vi "Periodic Tasks.vi"(8 "error in":errorcluster) -> ()   [LabVIEW 2016]
doc: "This VI runs in parallel to other tasks. It can contain as many user-defined periodic loops as you need. These can carry out PID or other sorts of timed response."
uses:
  <vilib>/Rock Robotics/SystemInterfaces/DIO/FPGA_DIOPWMChannel.ctl
  <vilib>/Rock Robotics/WPI/MotorControl/WPI_MotorControlOpen Victor.vi
  <vilib>/Rock Robotics/Network Tables/SD Write Number.vi
  <vilib>/addons/control/pid/pid.llb/PID Control Input Filter (DBL).vi
  <vilib>/addons/control/pid/pid.llb/PID (DBL).vi
  <vilib>/addons/control/pid/NI_PID_pid.lvlib
panel:
  in  "PID gains":T1={"proportional gain (Kc)"=0.1, "integral time (Ti, min)"=0.2, "derivative time (Td, min)"=0.0} {"derivative time (Td, min)" format="%.3f"; "integral time (Ti, min)" format="%.3f"; "proportional gain (Kc)" format="%.3f"}
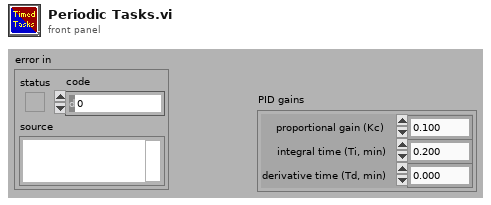
[diagram p1: front panel]
types:
  T1 = cluster{"proportional gain (Kc)":dbl, "integral time (Ti, min)":dbl, "derivative time (Td, min)":dbl}
  T2 = typedef "FPGA_DIOPWMChannel.ctl" = enum8{"PWM 0", "PWM 1", "PWM 2", "PWM 3", "PWM 4", "PWM 5", "PWM 6", "PWM 7", "PWM 8", "PWM 9", "PWM MXP 0", "PWM MXP 1", "PWM MXP 2", "PWM MXP 3", "PWM MXP 4", "PWM MXP 5", "PWM MXP 6", "PWM MXP 7", "PWM MXP 8", "PWM MXP 9", "Invalid"}
  T3 = typedef "WPI_MotorControlDeviceRef.ctl" = cluster{"DeviceStatus":errorcluster, "Type":T4, "PWM":cluster{"PWM Channel":T2, "DeadBand":T5}, "CAN":cluster{"Device Number":u8, "SetOutput VI Ref":variant, "GetOutput VI Ref":variant, "Enable VI Ref":variant, "Disable VI Ref":variant, "Data":variant}, "Invert":bool}
  T4 = typedef "WPI_MotorControlType.ctl" = enum16{"PWM", "CAN"}
  T5 = typedef "WPI_PWMDeadband.ctl" = cluster{"Name":string, "maxPositivePwm":i32, "minPositivePwm":i32, "centerPwm":i32, "maxNegativePwm":i32, "minNegativePwm":i32, "angularRange":u16}
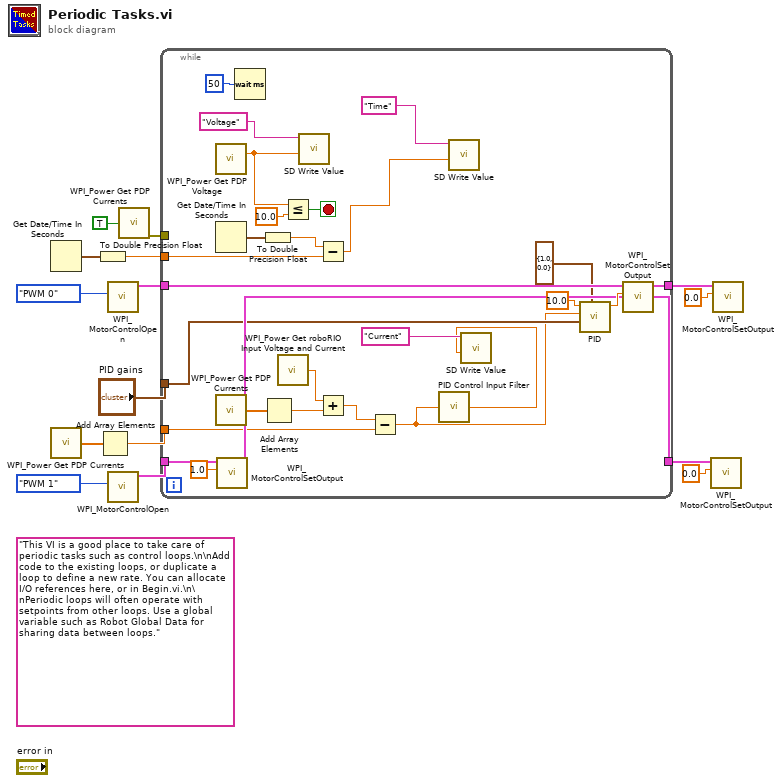
[diagram p0: block diagram]
diagram:
  (unwired) "This VI is a good place to take care of periodic tasks such as control loops.\n\nAdd code to the existing loops, or duplicate a loop to define a new rate. You can allocate I/O references here, or in Begin.vi.\n\nPeriodic loops will often operate with setpoints from other loops. Use a global variable such as Robot Global Data for sharing data between loops."
  n1 = Get Date/Time In Seconds() -> (seconds since 1Jan1904=w5:timestamp)
  n2 = call <vilib>:"WPI_Power Get PDP Currents.vi"() -> ("all currents (A)"=w2:dbl[])  [unwired: 13 in, 2 out]
  n3 = To Double Precision Float(number=w5) -> (double precision float=w4:dbl)
  n4 = Add Array Elements(numeric array=w2) -> (sum=w1:dbl)
  n5 = call-poly <vilib>:"WPI_MotorControlOpen.vi"("PWM Channel"=FPGA_DIOPWMChannel."PWM 0") -> ("MotorControlDeviceRef"=w11:T3)  [unwired: 9 in, 1 out]
  n6 = call-poly <vilib>:"WPI_MotorControlOpen.vi"("PWM Channel"=FPGA_DIOPWMChannel."PWM 1") -> ("MotorControlDeviceRef"=w10:T3)  [unwired: 9 in, 1 out]
  n7 = call <vilib>:"WPI_Power Get PDP Currents.vi"("Tare Currents?"=TRUE) -> ("error out"=w14:errorcluster)  [unwired: 12 in, 2 out]
  n8 = while {
    tunnel: w14 -> [_]
    tunnel: w11 -> [w36]
    tunnel: w10 -> [w37]
    tunnel: [w32] -> w9
    tunnel: [w31] -> w8
    tunnel: w4 -> [w27]
    tunnel: "PID gains" -> [w23]
    tunnel: w1 -> [w22]
    stop <- w33 stop-if-true
    n9 = call <vilib>:"WPI_Power Get PDP Voltage.vi"() -> ("voltage (V)"=w30:dbl)  [unwired: 14 in, 1 out]
    n10 = Get Date/Time In Seconds() -> (seconds since 1Jan1904=w29:timestamp)
    n11 = call <vilib>:"WPI_Power Get PDP Currents.vi"() -> ("all currents (A)"=w40:dbl[])  [unwired: 13 in, 2 out]
    n12 = call <vilib>:"WPI_MotorControlSetOutput.vi"("Output"=1.0, "MotorControlDevRef"=w37) -> ("MotorControlDevRef"=w31:T3)  [unwired: 7 in, 2 out]
    n13 = Wait (ms)(milliseconds to wait=u32 50) -> ()  [unwired: 1 out]
    n14 = To Double Precision Float(number=w29) -> (double precision float=w28:dbl)
    n15 = Add Array Elements(numeric array=w40) -> (sum=w38:dbl)
    n16 = call <vilib>:"WPI_Power Get roboRIO Input Voltage and Current.vi"() -> ("roboRIO input current (A)"=w39:dbl)  [unwired: 13 in, 2 out]
    n17 = Less Or Equal?(x=w30, y=10.0) -> (x <= y?=w33:bool)
    n18 = call-poly <vilib>:"SD Write Value.vi"("Numeric"=w30, "Name"="Voltage") -> ()  [unwired: 8 in, 2 out]
    n19 = Subtract(x=w28, y=w27) -> (x-y=w17:dbl)
    n20 = Add(x=w39, y=w38) -> (x+y=w21:dbl)
    n21 = Subtract(x=w21, y=w22) -> (x-y=w19:dbl)
    n22 = call-poly <vilib>:"PID Control Input Filter.vi"("input"=w19) -> ("output"=w18:dbl)  [unwired: 4 in]
    n23 = call-poly <vilib>:"SD Write Value.vi"("Numeric"=w17, "Name"="Time") -> ()  [unwired: 8 in, 2 out]
    n24 = call-poly <vilib>:"SD Write Value.vi"("Numeric"=w18, "Name"="Current") -> ()  [unwired: 8 in, 2 out]
    n25 = call-poly <vilib>:"PID.vi"("output range"=cluster{"output high":dbl, "output low":dbl} {"output high"=1.0, "output low"=0.0}, "PID gains"=w23, "process variable"=w19, "setpoint"=10.0) -> ("output"=w35:dbl)  [unwired: 6 in, 1 out]
    n26 = call <vilib>:"WPI_MotorControlSetOutput.vi"("Output"=w35, "MotorControlDevRef"=w36) -> ("MotorControlDevRef"=w32:T3)  [unwired: 7 in, 2 out]
  }
  n27 = call <vilib>:"WPI_MotorControlSetOutput.vi"("Output"=0.0, "MotorControlDevRef"=w8) -> ()  [unwired: 7 in, 3 out]
  n28 = call <vilib>:"WPI_MotorControlSetOutput.vi"("Output"=0.0, "MotorControlDevRef"=w9) -> ()  [unwired: 7 in, 3 out]
